vi "Calibration Parameters Menu.vi"() -> ()   [LabVIEW 2013]
panel:
  in  "Samples Per Sweep":dbl
  in  "Calibration Sample Rate":dbl
  in  "Number of Sweeps":dbl
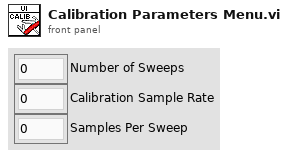
[diagram p1: front panel]
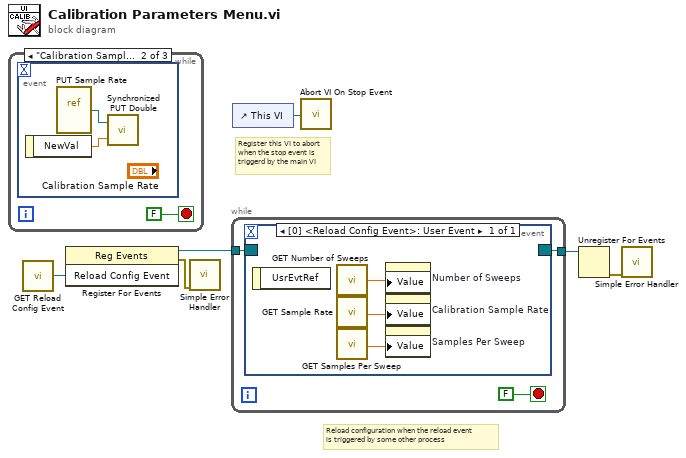
[diagram p0: block diagram]
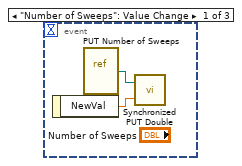
[diagram p2: hidden frame]
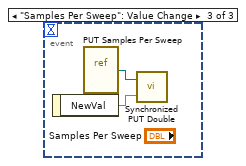
[diagram p3: hidden frame]
diagram:
  # "Reload configuration when the reload event\nis triggered by some other process"
  # "Register this VI to abort\nwhen the stop event is\ntriggerd by the main VI"
  n1 = while {
    stop <- FALSE stop-if-true
    n2 = event shown="[1] \"Calibration Sample Rate\": Value Change" {
      selector: _ -> [_ _ _]
      dyn-events: _ -> [_ _ _]
      timeout: _ -> [_ _ _]
      event "Number of Sweeps": Value Change {
        n3 = event-data() -> ("NewVal"=w8:dbl)  [unwired: 1 in]
        n4 = vi-ref "PUT Number of Sweeps.vi"() -> (w9:refnum<vi>)
        n5 = call "Synchronized PUT Double.vi"("PUT Value"=w8, "PUT VI Reference"=w9) -> ()  [unwired: 1 in]
      }
      event "Calibration Sample Rate": Value Change {
        n6 = event-data() -> ("NewVal"=w11:dbl)  [unwired: 1 in]
        n7 = vi-ref "PUT Sample Rate.vi"() -> (w10:refnum<vi>)
        n8 = call "Synchronized PUT Double.vi"("PUT Value"=w11, "PUT VI Reference"=w10) -> ()  [unwired: 1 in]
      }
      event "Samples Per Sweep": Value Change {
        n9 = event-data() -> ("NewVal"=w12:dbl)  [unwired: 1 in]
        n10 = vi-ref "PUT Samples Per Sweep.vi"() -> (w13:refnum<vi>)
        n11 = call "Synchronized PUT Double.vi"("PUT Value"=w12, "PUT VI Reference"=w13) -> ()  [unwired: 1 in]
      }
    }
  }
  n12 = call "GET Reload Config Event.vi"() -> ("Reload Config Event"=w1:refnum<user-event>)
  n13 = register-events(w1) -> (reference out=w2:refnum<event-registration>, error out=w3:errorcluster)  [unwired: 2 in]
  n14 = call <vilib>:"Simple Error Handler.vi"("error in (no error)"=w3) -> ()  [unwired: 4 in, 5 out]
  n15 = while {
    tunnel: [w16] -> w4
    tunnel: w2 -> [w15]
    stop <- FALSE stop-if-true
    n16 = event shown="[0] <Reload Config Event>: User Event" {
      selector: w15 -> [_]
      dyn-events: [_] -> w16
      timeout: _ -> [_]
      event User Event {
        n17 = event-data() -> ()  [unwired: 1 in, 1 out]
        n18 = call "GET Number of Sweeps.vi"() -> ("Number of Sweeps"=w19:dbl)
        n19 = call "GET Sample Rate.vi"() -> ("Calibration Sample Rate"=w18:dbl)
        n20 = call "GET Samples Per Sweep.vi"() -> ("Samples Per Sweep"=w17:dbl)
        n21 = property on="Number of Sweeps" class="DigNum (strict)"("Value"=w19) -> ()  [unwired: 2 in, 2 out]
        n22 = property on="Calibration Sample Rate" class="DigNum (strict)"("Value"=w18) -> ()  [unwired: 2 in, 2 out]
        n23 = property on="Samples Per Sweep" class="DigNum (strict)"("Value"=w17) -> ()  [unwired: 2 in, 2 out]
      }
    }
  }
  n24 = control-ref of="This VI"() -> (w6:refnum<vi>)
  n25 = call "Abort VI On Stop Event.vi"("VI Reference"=w6) -> ()
  n26 = Unregister For Events(event registration refnum=w4) -> (error out=w5:errorcluster)  [unwired: 1 in]
  n27 = call <vilib>:"Simple Error Handler.vi"("error in (no error)"=w5) -> ()  [unwired: 4 in, 5 out]
